vi "HRM-AQN-myDAQ_close.vi"(8 "error in (no error)":errorcluster, 11 "AQN cluster in":T1) -> (0 "error out":errorcluster)   [LabVIEW 2020]
uses:
  HRM-AQN-input_clust.ctl
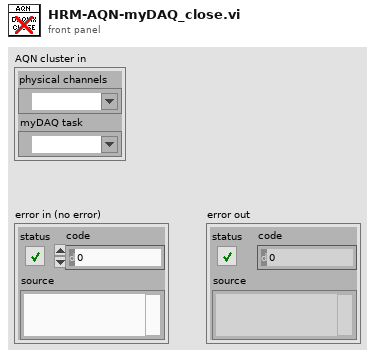
[diagram p1: front panel]
types:
  T1 = typedef "HRM-AQN-input_clust.ctl" = cluster{"physical channels":tag, "myDAQ task":refnum<k21>}
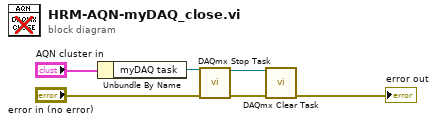
[diagram p0: block diagram]
diagram:
  n1 = Unbundle By Name("AQN cluster in") -> ("myDAQ task"=w5:refnum<k21>)
  n2 = call <vilib>:"DAQmx Stop Task.vi"("task/channels in"=w5, "error in"="error in (no error)") -> ("task out"=w2:refnum<k21>, "error out"=w3:errorcluster)  [unwired: 12 in]
  n3 = call <vilib>:"DAQmx Clear Task.vi"("task in"=w2, "error in"=w3) -> ("error out"=→"error out":errorcluster)  [unwired: 13 in]
